vi "Define.vi"(11 "Init Data":T1) -> (3 "Boolean out":refnum<class "Boolean.lvclass">)   [LabVIEW 2020, in "Conditum.lvlib" / "Columns.lvlib" / "Boolean.lvclass"]
uses:
  Boolean.lvclass
  C:/dev/lv20CE/lv-conditum/Conditum/Columns/Type/Type.lvclass
  Boolean Definition.ctl
  Type/Definition.ctl
  Attributes.ctl
  Definition.ctl
  Field Type.ctl
  Type/Type.lvclass/Type.ctl
  Boolean.lvclass/Boolean.ctl
  Type/Type.lvclass
  Conditum.lvlib
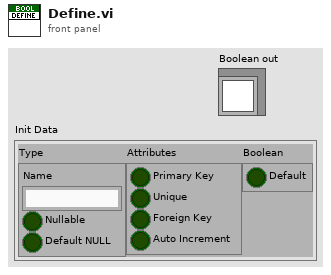
[diagram p1: front panel]
types:
  T1 = typedef "Conditum.lvlib/Columns.lvlib/Boolean.lvclass/Boolean Definition.ctl" = cluster{"Type":T2, "Attributes":T3, "Boolean":T4}
  T2 = typedef "Conditum.lvlib/Columns.lvlib/Type.lvclass/Definition.ctl" = cluster{"Name":string, "Nullable":bool, "Default NULL":bool}
  T3 = typedef "Conditum.lvlib/Attributes.ctl" = cluster{"Primary Key":bool, "Unique":bool, "Foreign Key":bool, "Auto Increment":bool}
  T4 = typedef "Conditum.lvlib/Columns.lvlib/Boolean.lvclass/Definition.ctl" = cluster{"Default":bool}
  T5 = typedef "Conditum.lvlib/Field Type.ctl" = enum16{"None", "ID", "Boolean", "Integer", "Double", "Timestamp", "String", "Text", "Entity"}
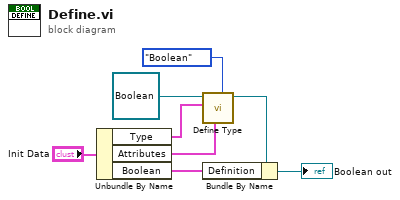
[diagram p0: block diagram]
diagram:
  n1 = Unbundle By Name("Init Data") -> ("Type"=w3:T2, "Attributes"=w2:T3, "Boolean"=w5:T4)
  n2 = call "Define Type.vi"("Type"=Field_Type."Boolean", "Attributes"=w2, "Definition"=w3, "Type in"=refnum<class "Boolean.lvclass"> refnum ("Boolean out")) -> ("Type out"=w4:refnum<class "Boolean.lvclass">)  [unwired: 7 in]
  n3 = Bundle By Name(cluster=w4, "Definition"=w5) -> (→"Boolean out":refnum<class "Boolean.lvclass">)
